vi "read channel scaling file.vi"(4 "include lab ambient? (T)":bool=TRUE, 6 "suppress inactive? (F)":bool, 9 "mode (all)":enum16{"all", "inputs", "outputs", "digital"}(ring), 11 "file path":path) -> (0 "channelTypeCount":i32[](array[numeric]), 1 "Total channels":i32, 2 "channelConfig":T1[](array[typedef]), 3 "activeChannelCount":u16, 5 "FIFO channels":u16)   [LabVIEW 2018]
uses:
  Type Defs/scalingMethods.ctl
  Type Defs/channelScalingTypes.ctl
  PC/type defs/channelControl.ctl
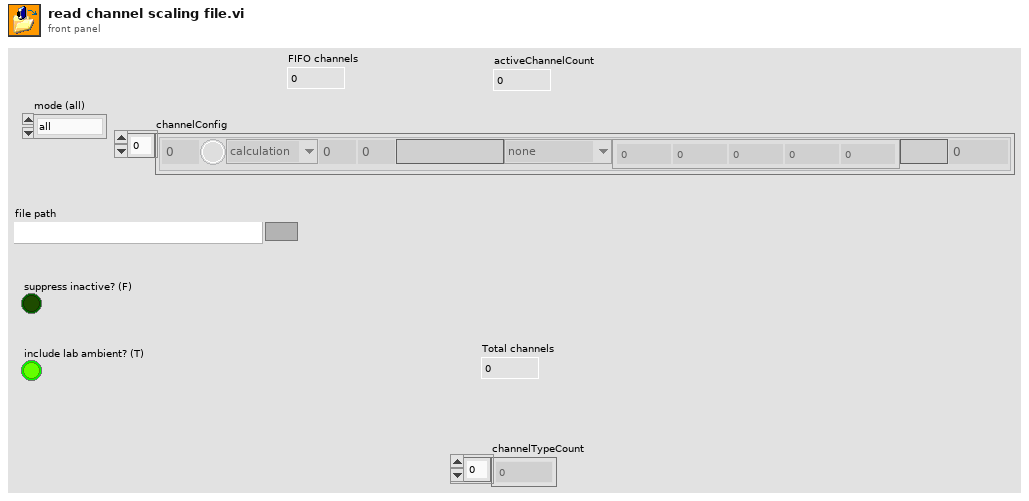
[diagram p1: front panel]
types:
  T1 = typedef "channelControl.ctl" = cluster{"index":u16, "active":bool, "channelType":T2, "module":u16, "terminal":u16, "channelName":string, "scalingMethod":T3, "scalingParameters":dbl[], "scaledUnits":string, "tempOffset":dbl}
  T2 = typedef "channelScalingTypes.ctl" = enum16{"calculation", "measurement", "scanivalve", "output", "digital"}
  T3 = typedef "scalingMethods.ctl" = enum16{"none", "linear", "thermocouple", "polynomial", "encoder", "RTD"}
  T4 = enum16{"open", "replace", "create", "open or create", "replace or create", "replace or create with confirmation"}
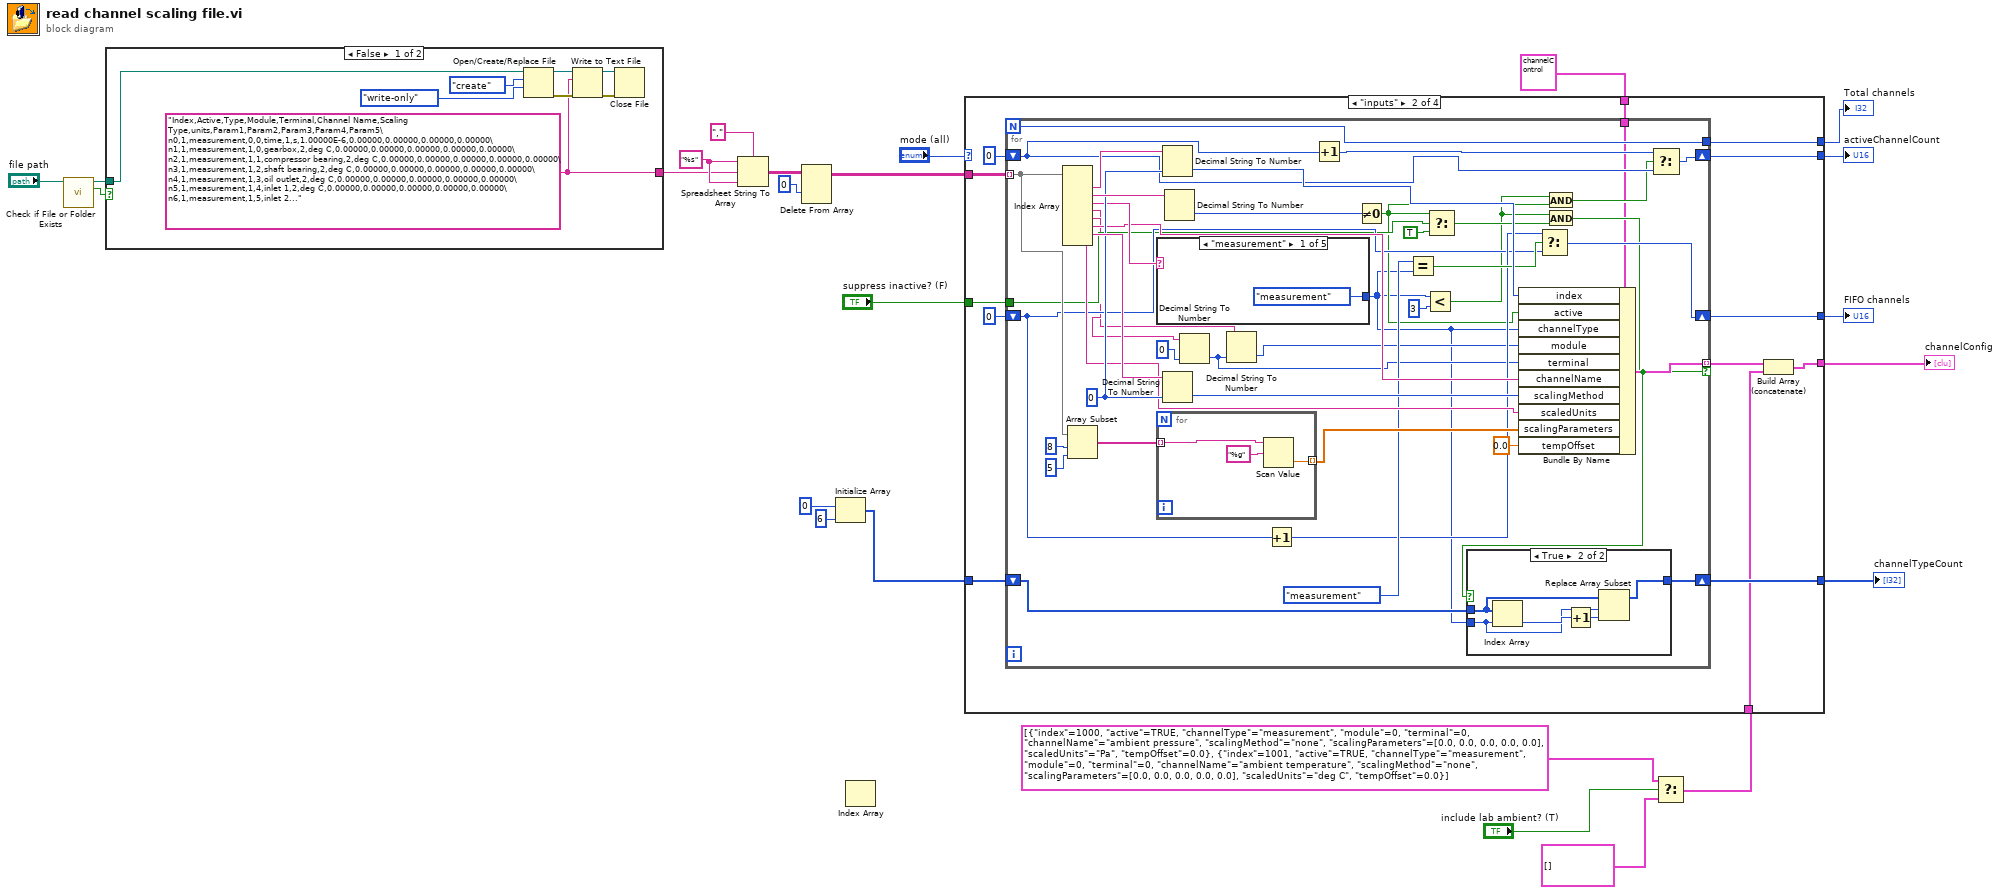
[diagram p0: block diagram]
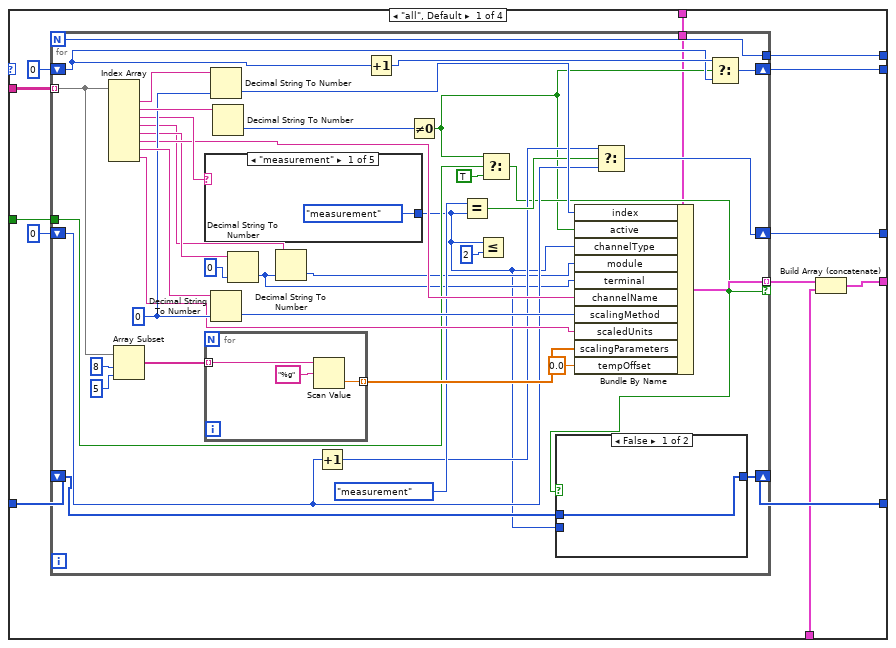
[diagram p2: hidden frame]
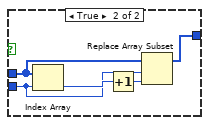
[diagram p3: hidden frame]
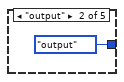
[diagram p4: hidden frame]
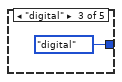
[diagram p5: hidden frame]
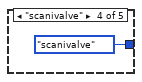
[diagram p6: hidden frame]
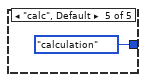
[diagram p7: hidden frame]
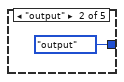
[diagram p9: hidden frame]
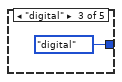
[diagram p10: hidden frame]
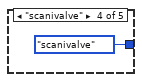
[diagram p11: hidden frame]
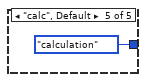
[diagram p12: hidden frame]
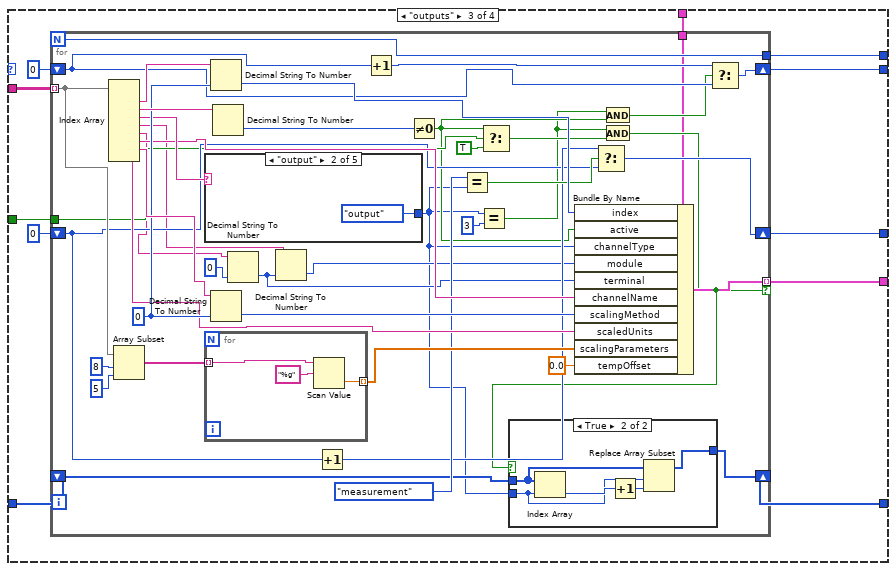
[diagram p13: hidden frame]
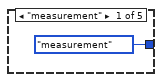
[diagram p15: hidden frame]
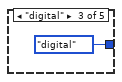
[diagram p16: hidden frame]
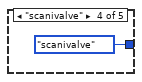
[diagram p17: hidden frame]
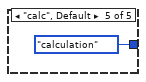
[diagram p18: hidden frame]
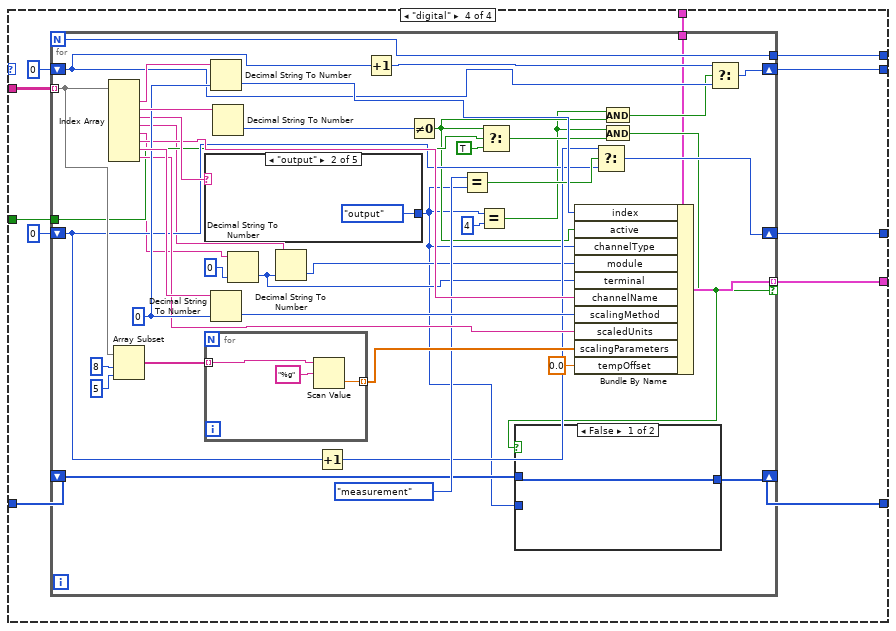
[diagram p19: hidden frame]
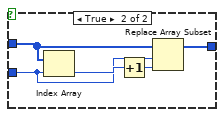
[diagram p20: hidden frame]
diagram:
  w19 = "%s" ("format string")
  n1 = call <vilib>:"Check if File or Folder Exists.vi"("path"="file path") -> ("file or folder exists?"=w18:bool, "dup path"=w17:path)  [unwired: 8 in, 1 out]
  n2 = case shown="False" w18 {
    tunnel: w17 -> [w26 w33]
    tunnel: [w25 w34] -> w15
    frame False {
      w25 = "Index,Active,Type,Module,Terminal,Channel Name,Scaling Type,units,Param1,Param2,Param3,Param4,Param5\n0,1,measurement,0,0,time,1,s,1.00000E-6,0.00000,0.00000,0.00000,0.00000\n1,1,measurement,1,0,gearbox,2,deg C,0.00000,0.00000,0.00000,0.00000,0.00000\n2,1,measurement,1,1,compressor bearing,2,deg C,0.00000,0.00000,0.00000,0.00000,0.00000\n3,1,measurement,1,2,shaft bearing,2,deg C,0.00000,0.00000,0.00000,0.00000,0.00000\n4,1,measurement,1,3,oil outlet,2,deg C,0.00000,0.00000,0.00000,0.00000,0.00000\n5,1,measurement,1,4,inlet 1,2,deg C,0.00000,0.00000,0.00000,0.00000,0.00000\n6,1,measurement,1,5,inlet 2,2,deg C,0.00000,0.00000,0.00000,0.00000,0.00000\n7,1,measurement,1,6,outlet 1,2,deg C,0.00000,0.00000,0.00000,0.00000,0.00000\n8,1,measurement,1,7,outlet 2,2,deg C,0.00000,0.00000,0.00000,0.00000,0.00000\n9,1,measurement,1,8,CJC_A,0,deg C,0.00000,0.00000,0.00000,0.00000,0.00000\n10,1,measurement,1,9,CJC_B,0,deg C,0.00000,0.00000,0.00000,0.00000,0.00000\n11,1,measurement,2,0,RTD_0,5,deg C,1.00000,0.00000,0.00000,0.00000,0.00000\n12,1,measurement,2,1,RTD_1,5,deg C,1.00000,0.00000,0.00000,0.00000,0.00000\n13,1,measurement,2,2,RTD_2,5,deg C,1.00000,0.00000,0.00000,0.00000,0.00000\n14,1,measurement,2,3,RTD_3,5,deg C,1.00000,0.00000,0.00000,0.00000,0.00000\n15,0,measurement,3,0,,0,,0.00000,0.00000,0.00000,0.00000,0.00000\n16,1,measurement,3,1,inlet pressure,1,bar,1405.20000,0.00000,0.00000,0.00000,0.00000\n17,1,measurement,3,2,outlet pressure,1,bar,2290.30000,0.00000,0.00000,0.00000,0.00000\n18,1,measurement,3,3,plenum pressure,1,bar,2326.30000,0.00000,0.00000,0.00000,0.00000\n19,1,measurement,4,0,Motor speed,1,RPM,74300.00000,0.00000,0.00000,0.00000,0.00000\n20,1,measurement,4,1,V-cone delta P,1,bar,37.50000,-4.00000,0.00000,0.00000,0.00000\n21,0,measurement,4,2,,0,,0.00000,0.00000,0.00000,0.00000,0.00000\n22,0,measurement,4,3,,0,,0.00000,0.00000,0.00000,0.00000,0.00000\n23,0,measurement,4,4,,0,,0.00000,0.00000,0.00000,0.00000,0.00000\n24,0,measurement,4,5,,0,,0.00000,0.00000,0.00000,0.00000,0.00000\n25,0,measurement,4,6,,0,,0.00000,0.00000,0.00000,0.00000,0.00000\n26,1,measurement,4,7,Motor power,1,W,5500.00000,0.00000,0.00000,0.00000,0.00000\n27,1,measurement,5,0,Accelerometer,1,m/s/s,98.10000,0.00000,0.00000,0.00000,0.00000\n28,1,measurement,5,1,,0,,0.00000,0.00000,0.00000,0.00000,0.00000\n29,1,measurement,5,2,,0,,0.00000,0.00000,0.00000,0.00000,0.00000\n30,1,measurement,5,3,,0,,0.00000,0.00000,0.00000,0.00000,0.00000\n31,1,measurement,5,4,,0,,0.00000,0.00000,0.00000,0.00000,0.00000\n32,1,measurement,5,5,,0,,0.00000,0.00000,0.00000,0.00000,0.00000\n33,1,measurement,5,6,Hotwire 1,3,,0.00000,0.00000,0.00000,0.00000,0.00000\n34,1,measurement,5,7,,0,,0.00000,0.00000,0.00000,0.00000,0.00000\n35,1,measurement,5,8,,0,,0.00000,0.00000,0.00000,0.00000,0.00000\n36,1,measurement,5,9,,0,,0.00000,0.00000,0.00000,0.00000,0.00000\n37,1,measurement,5,10,,0,,0.00000,0.00000,0.00000,0.00000,0.00000\n38,1,measurement,5,11,,0,,0.00000,0.00000,0.00000,0.00000,0.00000\n39,1,measurement,5,12,,0,,0.00000,0.00000,0.00000,0.00000,0.00000\n40,1,measurement,5,13,,0,,0.00000,0.00000,0.00000,0.00000,0.00000\n41,1,measurement,5,14,,0,,0.00000,0.00000,0.00000,0.00000,0.00000\n42,1,measurement,5,15,,0,,0.00000,0.00000,0.00000,0.00000,0.00000\n43,1,measurement,5,16,,0,,0.00000,0.00000,0.00000,0.00000,0.00000\n44,1,measurement,5,17,,0,,0.00000,0.00000,0.00000,0.00000,0.00000\n45,1,measurement,5,18,,0,,0.00000,0.00000,0.00000,0.00000,0.00000\n46,1,measurement,5,19,,0,,0.00000,0.00000,0.00000,0.00000,0.00000\n47,1,measurement,5,20,,0,,0.00000,0.00000,0.00000,0.00000,0.00000\n48,1,measurement,5,21,oil pressure,1,?,1.00000,0.00000,0.00000,0.00000,0.00000\n49,1,measurement,5,22,butterfly valve position,1,,0.00000,0.00000,0.00000,0.00000,0.00000\n50,1,measurement,5,23,ball valve position,1,,0.00000,0.00000,0.00000,0.00000,0.00000\n51,1,measurement,5,24,,0,,0.00000,0.00000,0.00000,0.00000,0.00000\n52,1,measurement,5,25,,0,,0.00000,0.00000,0.00000,0.00000,0.00000\n53,1,measurement,5,26,,0,,0.00000,0.00000,0.00000,0.00000,0.00000\n54,1,measurement,5,27,,0,,0.00000,0.00000,0.00000,0.00000,0.00000\n55,1,measurement,5,28,,0,,0.00000,0.00000,0.00000,0.00000,0.00000\n56,1,measurement,5,29,,0,,0.00000,0.00000,0.00000,0.00000,0.00000\n57,1,measurement,5,30,,0,,0.00000,0.00000,0.00000,0.00000,0.00000\n58,1,measurement,5,31,,0,,0.00000,0.00000,0.00000,0.00000,0.00000\n59,1,output,6,0,ball valve drive,1,%,-10.00000,10.00000,0.00000,0.00000,0.00000\n60,1,output,6,1,,0,,0.00000,0.00000,0.00000,0.00000,0.00000\n61,1,output,6,2,,0,,0.00000,0.00000,0.00000,0.00000,0.00000\n62,1,output,6,3,butterfly valve drive,1,%,-10.00000,10.00000,0.00000,0.00000,0.00000\n63,1,digital,7,0,,0,,0.00000,0.00000,0.00000,0.00000,0.00000\n64,1,digital,7,1,,0,,0.00000,0.00000,0.00000,0.00000,0.00000\n65,1,digital,7,2,,0,,0.00000,0.00000,0.00000,0.00000,0.00000\n66,1,digital,7,3,shaft encoder,4,RPM,8.00000,0.00000,0.00000,0.00000,0.00000\n67,1,digital,7,4,e-stop,0,,0.00000,0.00000,0.00000,0.00000,0.00000\n68,1,digital,7,5,,0,,0.00000,0.00000,0.00000,0.00000,0.00000\n69,1,digital,7,6,,0,,0.00000,0.00000,0.00000,0.00000,0.00000\n70,1,digital,7,7,pulsator encoder,4,RPM,1.00000,0.00000,0.00000,0.00000,0.00000\n71,1,digital,8,0,,0,,0.00000,0.00000,0.00000,0.00000,0.00000\n72,1,digital,8,1,,0,,0.00000,0.00000,0.00000,0.00000,0.00000\n73,1,digital,8,2,,0,,0.00000,0.00000,0.00000,0.00000,0.00000\n74,1,digital,8,3,,0,,0.00000,0.00000,0.00000,0.00000,0.00000\n75,1,digital,8,4,,0,,0.00000,0.00000,0.00000,0.00000,0.00000\n76,1,digital,8,5,,0,,0.00000,0.00000,0.00000,0.00000,0.00000\n77,1,digital,8,6,,0,,0.00000,0.00000,0.00000,0.00000,0.00000\n78,1,digital,8,7,,0,,0.00000,0.00000,0.00000,0.00000,0.00000\n79,0,measurement,/,,Torque encoder,4,RPM,39.00000,0.00000,0.00000,0.00000,0.00000\n80,0,measurement,/,,Torque phase,0,,0.00000,0.00000,0.00000,0.00000,0.00000\n81,1,measurement,/,,pulsator encoder,4,ROM,1.00000,0.00000,0.00000,0.00000,0.00000\n" ("defaultChannelConfigFile")
      n3 = Open/Create/Replace File(file path (use dialog)=w26, operation (0:open)=T4."create", access (0:read/write)=enum16{"read/write", "read-only", "write-only"}."write-only") -> (refnum out=w31:refnum<file>, error out=w32:errorcluster)  [unwired: 3 in, 1 out]
      n4 = Write to Text File(file (use dialog)=w31, text=w25, error in=w32) -> (refnum out=w29:refnum<file>, error out=w30:errorcluster)  [unwired: 1 in, 1 out]
      n5 = Close File(refnum=w29, error in=w30) -> ()  [unwired: 2 out]
    }
    frame True {
      n6 = Open/Create/Replace File(file path (use dialog)=w33, access (0:read/write)=enum16{"read/write", "read-only", "write-only"}."read-only") -> (refnum out=w38:refnum<file>, error out=w39:errorcluster)  [unwired: 4 in, 1 out]
      n7 = Read from Text File(file (use dialog)=w38, error in=w39) -> (refnum out=w36:refnum<file>, text=w34:string, error out=w37:errorcluster)  [unwired: 2 in, 1 out]
      n8 = Close File(refnum=w36, error in=w37) -> ()  [unwired: 2 out]
    }
  }
  n9 = Spreadsheet String To Array(delimiter (Tab)=",", format string=w19, spreadsheet string=w15, array type (2D Dbl)=w19) -> (array=w21:string[][])
  n10 = Delete From Array(array=w21, index (row)=0) -> (array with subset deleted=w23:string[][])  [unwired: 2 in, 1 out]
  n11 = Initialize Array(0, 6 ("dimension size")) -> (w8:i32[])
  n12 = Index Array() -> ()  [unwired: 2 in, 1 out]
  n13 = Select(t=T1[] [{"index"=1000, "active"=TRUE, "channelType"=enum."measurement", "module"=0, "terminal"=0, "channelName"="ambient pressure", "scalingMethod"=enum."none", "scalingParameters"=[0.0, 0.0, 0.0, 0.0, 0.0], "scaledUnits"="Pa", "tempOffset"=0.0}, {"index"=1001, "active"=TRUE, "channelType"=enum."measurement", "module"=0, "terminal"=0, "channelName"="ambient temperature", "scalingMethod"=enum."none", "scalingParameters"=[0.0, 0.0, 0.0, 0.0, 0.0], "scaledUnits"="deg C", "tempOffset"=0.0}] ("Array"), s="include lab ambient? (T)", f=T1[] []) -> (s? t:f=w2:T1[])
  n14 = case shown="\"inputs\"" "mode (all)" {
    tunnel: [w52 w119 w187 w255] -> w24
    tunnel: [w41 w108 w185 w253] -> w5
    tunnel: w23 -> [w49 w116 w184 w252]
    tunnel: [w47 w114 w182 w250] -> w14
    tunnel: [w46 w113 w181 w249] -> w13
    tunnel: "suppress inactive? (F)" -> [w45 w112 w180 w248]
    tunnel: w8 -> [w44 w111 w179 w246]
    tunnel: [w43 w110 w178 w247] -> w7
    tunnel: T1 {"index"=0, "active"=FALSE, "channelType"=enum."calculation", "module"=0, "terminal"=0, "channelName"="", "scalingMethod"=enum."none", "scalingParameters"=[], "scaledUnits"="", "tempOffset"=0.0} ("channelScaling") -> [w42 w109 w177 w245]
    tunnel: w2 -> [w40 w107 _ _]
    frame "all", Default {
      n15 = for {
        N -> [w67]
        tunnel: w49 -> [w84] mode=indexing
        tunnel: [w91] -> w50 mode=indexing if=w56
        shift-right: [w77] -> w52
        shift-left: u16 0 -> [w78]
        shift-right: [w68] -> w47
        shift-left: u16 0 -> [w69]
        tunnel: [w67] -> w46
        tunnel: w45 -> [w66]
        shift-right: [w57] -> w43
        shift-left: w44 -> [w59]
        tunnel: w42 -> [w54]
        w86 = u16 0
        n16 = Index Array(array=w84) -> (element #1=w90:string, element #2=w92:string, element #3=w75:string, element #4=w62:string, element #5=w63:string, element #6=w74:string, element #7=w87:string, element #8=w73:string)  [unwired: 8 in]
        n17 = Array Subset(array=w84, index=8, length=5) -> (w81:string[])
        n18 = case shown="\"measurement\"" w75 {
          tunnel: [channelScalingTypes."measurement" ("channelType") channelScalingTypes."output" ("channelType") channelScalingTypes."digital" ("channelType") channelScalingTypes."scanivalve" ("channelType") channelScalingTypes."calculation" ("channelType")] -> w58
          frame "measurement" {
          }
          frame "output" {
          }
          frame "digital" {
          }
          frame "scanivalve" {
          }
          frame "calc", Default {
          }
        }
        n19 = for {
          tunnel: w81 -> [w106] mode=indexing
          tunnel: [w104] -> w80 mode=indexing
          n20 = Scan Value(string=w106, format string="%g") -> (value=w104:dbl)  [unwired: 1 in, 1 out]
        }
        n21 = Decimal String To Number(string=w90, default (0L)=w86) -> (number=w89:u16)  [unwired: 1 in, 1 out]
        n22 = Decimal String To Number(string=w87, default (0L)=w86) -> (number=w85:u16)  [unwired: 1 in, 1 out]
        n23 = Decimal String To Number(string=w92) -> (number=w88:i32)  [unwired: 2 in, 1 out]
        n24 = Decimal String To Number(string=w63, default (0L)=u16 0 ("default (0 I32)")) -> (number=w61:u16)  [unwired: 1 in, 1 out]
        n25 = Decimal String To Number(string=w62, default (0L)=w61) -> (number=w60:u16)  [unwired: 1 in, 1 out]
        n26 = Increment(x=w69) -> (x+1=w70:u16)
        n27 = Increment(x=w78) -> (x+1=w79:u16)
        n28 = Not Equal To 0?(x=w88) -> (x != 0?=w55:bool)
        n29 = Equal?(x=channelScalingTypes."measurement", y=w58) -> (x = y?=w71:bool)
        n30 = Less Or Equal?(x=w58, y=u16 2) -> ()  [unwired: 1 out]
        n31 = Select(t=w55, s=w66, f=TRUE ("suppress inactive? (F)")) -> (s? t:f=w56:bool)
        n32 = case shown="False" w56 {
          tunnel: w59 -> [w93 w96]
          tunnel: w58 -> [_ w95]
          tunnel: [w93 w94] -> w57
          frame False {
          }
          frame True {
            n33 = Index Array(array=w96, index=w95) -> (element=w98:i32)
            n34 = Increment(x=w98) -> (x+1=w97:i32)
            n35 = Replace Array Subset(array=w96, new element=w97, index=w95) -> (w94:i32[])
          }
        }
        n36 = Bundle By Name(cluster=w54, "index"=w89, "active"=w55, "channelType"=w58, "module"=w60, "terminal"=w61, "channelName"=w74, "scalingMethod"=w85, "scaledUnits"=w73, "scalingParameters"=w80, "tempOffset"=0.0) -> (w91:T1)
        n37 = Select(t=w70, s=w71, f=w69) -> (s? t:f=w68:u16)
        n38 = Select(t=w79, s=w55, f=w78) -> (s? t:f=w77:u16)
      }
      n39 = Build Array (concatenate)(w50, w40) -> (w41:T1[])
    }
    frame "inputs" {
      n40 = for {
        N -> [w136]
        tunnel: w116 -> [w154] mode=indexing
        tunnel: [w161] -> w117 mode=indexing if=w122
        shift-right: [w147] -> w119
        shift-left: u16 0 -> [w148]
        shift-right: [w137] -> w114
        shift-left: u16 0 -> [w138]
        tunnel: [w136] -> w113
        tunnel: w112 -> [w135]
        shift-right: [w123] -> w110
        shift-left: w111 -> [w125]
        tunnel: w109 -> [w121]
        w156 = u16 0
        n41 = Index Array(array=w154) -> (element #1=w160:string, element #2=w162:string, element #3=w144:string, element #4=w129:string, element #5=w130:string, element #6=w143:string, element #7=w157:string, element #8=w142:string)  [unwired: 8 in]
        n42 = Array Subset(array=w154, index=8, length=5) -> (w151:string[])
        n43 = case shown="\"measurement\"" w144 {
          tunnel: [channelScalingTypes."measurement" ("channelType") channelScalingTypes."output" ("channelType") channelScalingTypes."digital" ("channelType") channelScalingTypes."scanivalve" ("channelType") channelScalingTypes."calculation" ("channelType")] -> w124
          frame "measurement" {
          }
          frame "output" {
          }
          frame "digital" {
          }
          frame "scanivalve" {
          }
          frame "calc", Default {
          }
        }
        n44 = for {
          tunnel: w151 -> [w176] mode=indexing
          tunnel: [w174] -> w150 mode=indexing
          n45 = Scan Value(string=w176, format string="%g") -> (value=w174:dbl)  [unwired: 1 in, 1 out]
        }
        n46 = Decimal String To Number(string=w160, default (0L)=w156) -> (number=w159:u16)  [unwired: 1 in, 1 out]
        n47 = Decimal String To Number(string=w157, default (0L)=w156) -> (number=w155:u16)  [unwired: 1 in, 1 out]
        n48 = Decimal String To Number(string=w162) -> (number=w158:i32)  [unwired: 2 in, 1 out]
        n49 = Decimal String To Number(string=w130, default (0L)=u16 0 ("default (0 I32)")) -> (number=w127:u16)  [unwired: 1 in, 1 out]
        n50 = Decimal String To Number(string=w129, default (0L)=w127) -> (number=w126:u16)  [unwired: 1 in, 1 out]
        n51 = Increment(x=w138) -> (x+1=w139:u16)
        n52 = Increment(x=w148) -> (x+1=w149:u16)
        n53 = Not Equal To 0?(x=w158) -> (x != 0?=w133:bool)
        n54 = Equal?(x=channelScalingTypes."measurement", y=w124) -> (x = y?=w140:bool)
        n55 = Less?(x=w124, y=u16 3) -> (x < y?=w131:bool)
        n56 = Select(t=w133, s=w135, f=TRUE ("suppress inactive? (F)")) -> (s? t:f=w132:bool)
        n57 = Bundle By Name(cluster=w121, "index"=w159, "active"=w133, "channelType"=w124, "module"=w126, "terminal"=w127, "channelName"=w143, "scalingMethod"=w155, "scaledUnits"=w142, "scalingParameters"=w150, "tempOffset"=0.0) -> (w161:T1)
        n58 = Select(t=w139, s=w140, f=w138) -> (s? t:f=w137:u16)
        n59 = And(x=w131, y=w133) -> (x .and. y?=w145:bool)
        n60 = And(x=w131, y=w132) -> (x .and. y?=w122:bool)
        n61 = case shown="True" w122 {
          tunnel: w125 -> [w163 w166]
          tunnel: w124 -> [_ w165]
          tunnel: [w163 w164] -> w123
          frame False {
          }
          frame True {
            n62 = Index Array(array=w166, index=w165) -> (element=w168:i32)
            n63 = Increment(x=w168) -> (x+1=w167:i32)
            n64 = Replace Array Subset(array=w166, new element=w167, index=w165) -> (w164:i32[])
          }
        }
        n65 = Select(t=w149, s=w145, f=w148) -> (s? t:f=w147:u16)
      }
      n66 = Build Array (concatenate)(w117, w107) -> (w108:T1[])
    }
    frame "outputs" {
      n67 = for {
        N -> [w204]
        tunnel: w184 -> [w222] mode=indexing
        tunnel: [w229] -> w185 mode=indexing if=w190
        shift-right: [w215] -> w187
        shift-left: u16 0 -> [w216]
        shift-right: [w205] -> w182
        shift-left: u16 0 -> [w206]
        tunnel: [w204] -> w181
        tunnel: w180 -> [w203]
        shift-right: [w191] -> w178
        shift-left: w179 -> [w193]
        tunnel: w177 -> [w189]
        w224 = u16 0
        n68 = Index Array(array=w222) -> (element #1=w228:string, element #2=w230:string, element #3=w212:string, element #4=w197:string, element #5=w198:string, element #6=w211:string, element #7=w225:string, element #8=w210:string)  [unwired: 8 in]
        n69 = Array Subset(array=w222, index=8, length=5) -> (w219:string[])
        n70 = case shown="\"output\"" w212 {
          tunnel: [channelScalingTypes."measurement" ("channelType") channelScalingTypes."output" ("channelType") channelScalingTypes."digital" ("channelType") channelScalingTypes."scanivalve" ("channelType") channelScalingTypes."calculation" ("channelType")] -> w192
          frame "measurement" {
          }
          frame "output" {
          }
          frame "digital" {
          }
          frame "scanivalve" {
          }
          frame "calc", Default {
          }
        }
        n71 = for {
          tunnel: w219 -> [w244] mode=indexing
          tunnel: [w242] -> w218 mode=indexing
          n72 = Scan Value(string=w244, format string="%g") -> (value=w242:dbl)  [unwired: 1 in, 1 out]
        }
        n73 = Decimal String To Number(string=w228, default (0L)=w224) -> (number=w227:u16)  [unwired: 1 in, 1 out]
        n74 = Decimal String To Number(string=w225, default (0L)=w224) -> (number=w223:u16)  [unwired: 1 in, 1 out]
        n75 = Decimal String To Number(string=w230) -> (number=w226:i32)  [unwired: 2 in, 1 out]
        n76 = Decimal String To Number(string=w198, default (0L)=u16 0 ("default (0 I32)")) -> (number=w195:u16)  [unwired: 1 in, 1 out]
        n77 = Decimal String To Number(string=w197, default (0L)=w195) -> (number=w194:u16)  [unwired: 1 in, 1 out]
        n78 = Increment(x=w206) -> (x+1=w207:u16)
        n79 = Increment(x=w216) -> (x+1=w217:u16)
        n80 = Not Equal To 0?(x=w226) -> (x != 0?=w201:bool)
        n81 = Equal?(x=channelScalingTypes."measurement", y=w192) -> (x = y?=w208:bool)
        n82 = Equal?(x=w192, y=u16 3) -> (x = y?=w199:bool)
        n83 = Select(t=w201, s=w203, f=TRUE ("suppress inactive? (F)")) -> (s? t:f=w200:bool)
        n84 = Bundle By Name(cluster=w189, "index"=w227, "active"=w201, "channelType"=w192, "module"=w194, "terminal"=w195, "channelName"=w211, "scalingMethod"=w223, "scaledUnits"=w210, "scalingParameters"=w218, "tempOffset"=0.0) -> (w229:T1)
        n85 = Select(t=w207, s=w208, f=w206) -> (s? t:f=w205:u16)
        n86 = And(x=w199, y=w201) -> (x .and. y?=w213:bool)
        n87 = And(x=w199, y=w200) -> (x .and. y?=w190:bool)
        n88 = case shown="True" w190 {
          tunnel: w193 -> [w231 w234]
          tunnel: w192 -> [_ w233]
          tunnel: [w231 w232] -> w191
          frame False {
          }
          frame True {
            n89 = Index Array(array=w234, index=w233) -> (element=w236:i32)
            n90 = Increment(x=w236) -> (x+1=w235:i32)
            n91 = Replace Array Subset(array=w234, new element=w235, index=w233) -> (w232:i32[])
          }
        }
        n92 = Select(t=w217, s=w213, f=w216) -> (s? t:f=w215:u16)
      }
    }
    frame "digital" {
      n93 = for {
        N -> [w272]
        tunnel: w252 -> [w290] mode=indexing
        tunnel: [w297] -> w253 mode=indexing if=w258
        shift-right: [w283] -> w255
        shift-left: u16 0 -> [w284]
        shift-right: [w273] -> w250
        shift-left: u16 0 -> [w274]
        tunnel: [w272] -> w249
        tunnel: w248 -> [w271]
        shift-right: [w261] -> w247
        shift-left: w246 -> [w260]
        tunnel: w245 -> [w257]
        w292 = u16 0
        n94 = Index Array(array=w290) -> (element #1=w296:string, element #2=w298:string, element #3=w280:string, element #4=w266:string, element #5=w265:string, element #6=w279:string, element #7=w293:string, element #8=w278:string)  [unwired: 8 in]
        n95 = Array Subset(array=w290, index=8, length=5) -> (w287:string[])
        n96 = case shown="\"output\"" w280 {
          tunnel: [channelScalingTypes."measurement" ("channelType") channelScalingTypes."output" ("channelType") channelScalingTypes."digital" ("channelType") channelScalingTypes."scanivalve" ("channelType") channelScalingTypes."calculation" ("channelType")] -> w259
          frame "measurement" {
          }
          frame "output" {
          }
          frame "digital" {
          }
          frame "scanivalve" {
          }
          frame "calc", Default {
          }
        }
        n97 = for {
          tunnel: w287 -> [w312] mode=indexing
          tunnel: [w310] -> w286 mode=indexing
          n98 = Scan Value(string=w312, format string="%g") -> (value=w310:dbl)  [unwired: 1 in, 1 out]
        }
        n99 = Decimal String To Number(string=w296, default (0L)=w292) -> (number=w295:u16)  [unwired: 1 in, 1 out]
        n100 = Decimal String To Number(string=w293, default (0L)=w292) -> (number=w291:u16)  [unwired: 1 in, 1 out]
        n101 = Decimal String To Number(string=w298) -> (number=w294:i32)  [unwired: 2 in, 1 out]
        n102 = Decimal String To Number(string=w265, default (0L)=u16 0 ("default (0 I32)")) -> (number=w262:u16)  [unwired: 1 in, 1 out]
        n103 = Decimal String To Number(string=w266, default (0L)=w262) -> (number=w264:u16)  [unwired: 1 in, 1 out]
        n104 = Increment(x=w274) -> (x+1=w275:u16)
        n105 = Increment(x=w284) -> (x+1=w285:u16)
        n106 = Not Equal To 0?(x=w294) -> (x != 0?=w269:bool)
        n107 = Equal?(x=channelScalingTypes."measurement", y=w259) -> (x = y?=w276:bool)
        n108 = Equal?(x=w259, y=u16 4) -> (x = y?=w267:bool)
        n109 = Select(t=w269, s=w271, f=TRUE ("suppress inactive? (F)")) -> (s? t:f=w268:bool)
        n110 = Bundle By Name(cluster=w257, "index"=w295, "active"=w269, "channelType"=w259, "module"=w264, "terminal"=w262, "channelName"=w279, "scalingMethod"=w291, "scaledUnits"=w278, "scalingParameters"=w286, "tempOffset"=0.0) -> (w297:T1)
        n111 = Select(t=w275, s=w276, f=w274) -> (s? t:f=w273:u16)
        n112 = And(x=w267, y=w269) -> (x .and. y?=w281:bool)
        n113 = And(x=w267, y=w268) -> (x .and. y?=w258:bool)
        n114 = case shown="False" w258 {
          tunnel: [w299 w302] -> w261
          tunnel: w260 -> [w299 w301]
          tunnel: w259 -> [_ w300]
          frame False {
          }
          frame True {
            n115 = Index Array(array=w301, index=w300) -> (element=w304:i32)
            n116 = Increment(x=w304) -> (x+1=w303:i32)
            n117 = Replace Array Subset(array=w301, new element=w303, index=w300) -> (w302:i32[])
          }
        }
        n118 = Select(t=w285, s=w281, f=w284) -> (s? t:f=w283:u16)
      }
    }
  }
  "activeChannelCount" <- w24
  "channelConfig" <- w5
  "FIFO channels" <- w14
  "Total channels" <- w13
  "channelTypeCount" <- w7
